vi "Plant Simulator in Engineering Units.vi"(6 "Initialize ?":bool, 8 "Sampling Time dt (s)":dbl, 10 "process parameters":T1={"static gain"=2.5, "lag (min)"=0.3, "dead cycles"=1, "load %"=40.0, "deadband"=2.0, "noise level %"=0.25, "initial PV"=0.0} {"initial PV" format="%.2f"; "noise level %" format="%.2f"; "lag (min)" format="%.2f"; "dead cycles" format="%.2f"; "deadband" format="%.1f"; "load %" format="%.2f"; "static gain" format="%.2f"}, 11 "Plnat Input (EGU)":dbl) -> (3 "Plant Output (EGU)":dbl)   [LabVIEW 2023]
uses:
  <vilib>/addons/control/pid/pid.llb/PID EGU to Percentage (DBL).vi
  <vilib>/addons/control/pid/pid.llb/PID Percentage to EGU (DBL).vi
  <vilib>/addons/control/pid/NI_PID_pid.lvlib
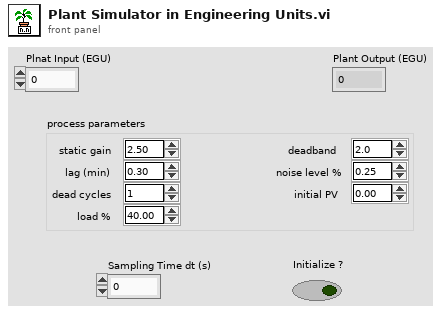
[diagram p1: front panel]
types:
  T1 = cluster{"static gain":dbl, "lag (min)":dbl, "dead cycles":i32, "load %":dbl, "deadband":dbl, "noise level %":dbl, "initial PV":dbl}
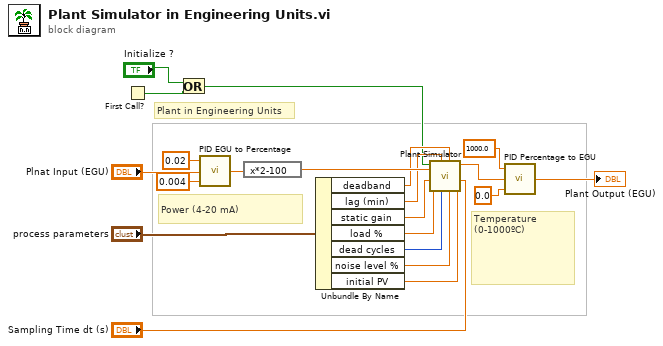
[diagram p0: block diagram]
diagram:
  # "Temperature \n(0-1000ºC)"
  # "Power (4-20 mA)"
  # "Plant in Engineering Units"
  n1 = First Call?() -> (First Call?: T/F=w3:bool)
  n2 = Or(x="Initialize ?", y=w3) -> (x .or. y?=w1:bool)
  n3 = call-poly <vilib>:"PID EGU to Percentage.vi"("minimum (EGU)"=0.004, "input (EGU)"="Plnat Input (EGU)", "maximum (EGU)"=0.02) -> ("% span"=w19:dbl)
  n4 = expression code="x*2-100"(w19) -> (w20:dbl)
  n5 = Unbundle By Name("process parameters") -> ("deadband"=w5:dbl, "lag (min)"=w10:dbl, "static gain"=w6:dbl, "load %"=w7:dbl, "dead cycles"=w4:i32, "noise level %"=w9:dbl, "initial PV"=w11:dbl)
  n6 = call "Plant Simulator.vi"("Initial PV"=w11, "dt (s)"="Sampling Time dt (s)", "Controller Noise (%)"=w9, "Valve Deadband"=w5, "Process Deadtime"=w4, "Lag (min)"=w10, "Process Load"=w7, "Process Gain"=w6, "Manipulated Variable (Output, %)"=w20, "Reinitialize"=w1) -> ("Process Variable (%)"=w13:dbl)  [unwired: 1 in]
  n7 = call-poly <vilib>:"PID Percentage to EGU.vi"("minimum (EGU)"=0.0, "% span"=w13, "maximum (EGU)"=1000.0) -> ("output (EGU)"=→"Plant Output (EGU)":dbl)  [unwired: 1 in]
